vi "ReversedEngineering FilterClassSearch.vi"(0 "dependencyClassPath":path[](array[path]), 2 "LoopIteration":i32, 4 "IgnoreClasses":path[](array[path]), 5 "error in (no error)":errorcluster, 6 "SerachDirs":path[](array[path]), 7 "Only Create this/these classes and its dependencis":bool, 8 "SearchOnlyClasses":bool, 9 "Only analyse this class methods and attributes(False)":bool, 10 "SearchOnlyTopVIs":bool, 11 "SyncOption":T1) -> (14 "dependencyClassPathOut":path[](array[path]), 15 "AnalyseClass":bool, 16 "AnalyseDone":bool, 17 "ClassPathToAnalyse":path, 19 "error out":errorcluster)   [LabVIEW 2012]
uses:
  <resource>/Framework/Providers/Open_GDS/UML/UMLEditor/UMLEditor_SyncOptions.ctl
  <resource>/Framework/Providers/Open_GDS/UML/UmlEditor_class/UmlEditor.lvclass
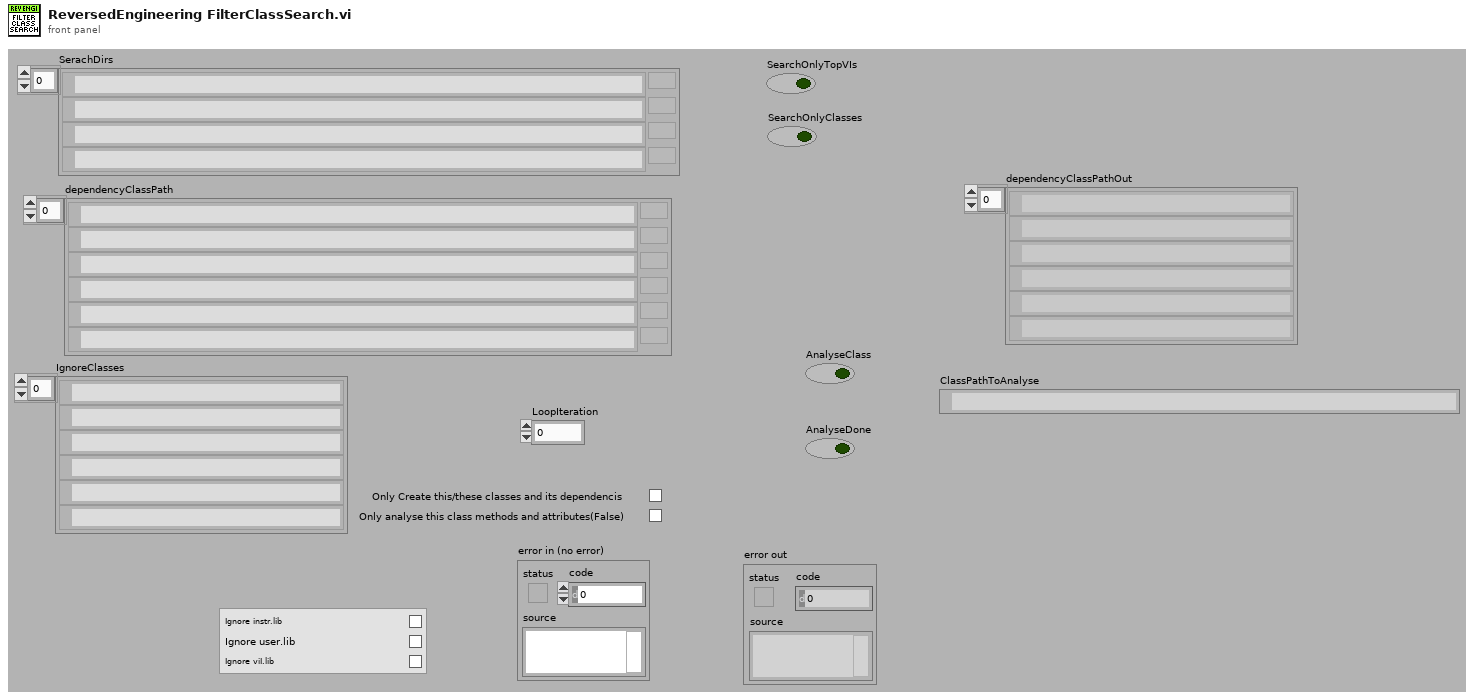
[diagram p1: front panel]
types:
  T1 = typedef "UMLEditor_SyncOptions.ctl" = cluster{"IgnoreInstrLib":bool, "IgnoreUserLib":bool, "IgnoreViLib":bool}
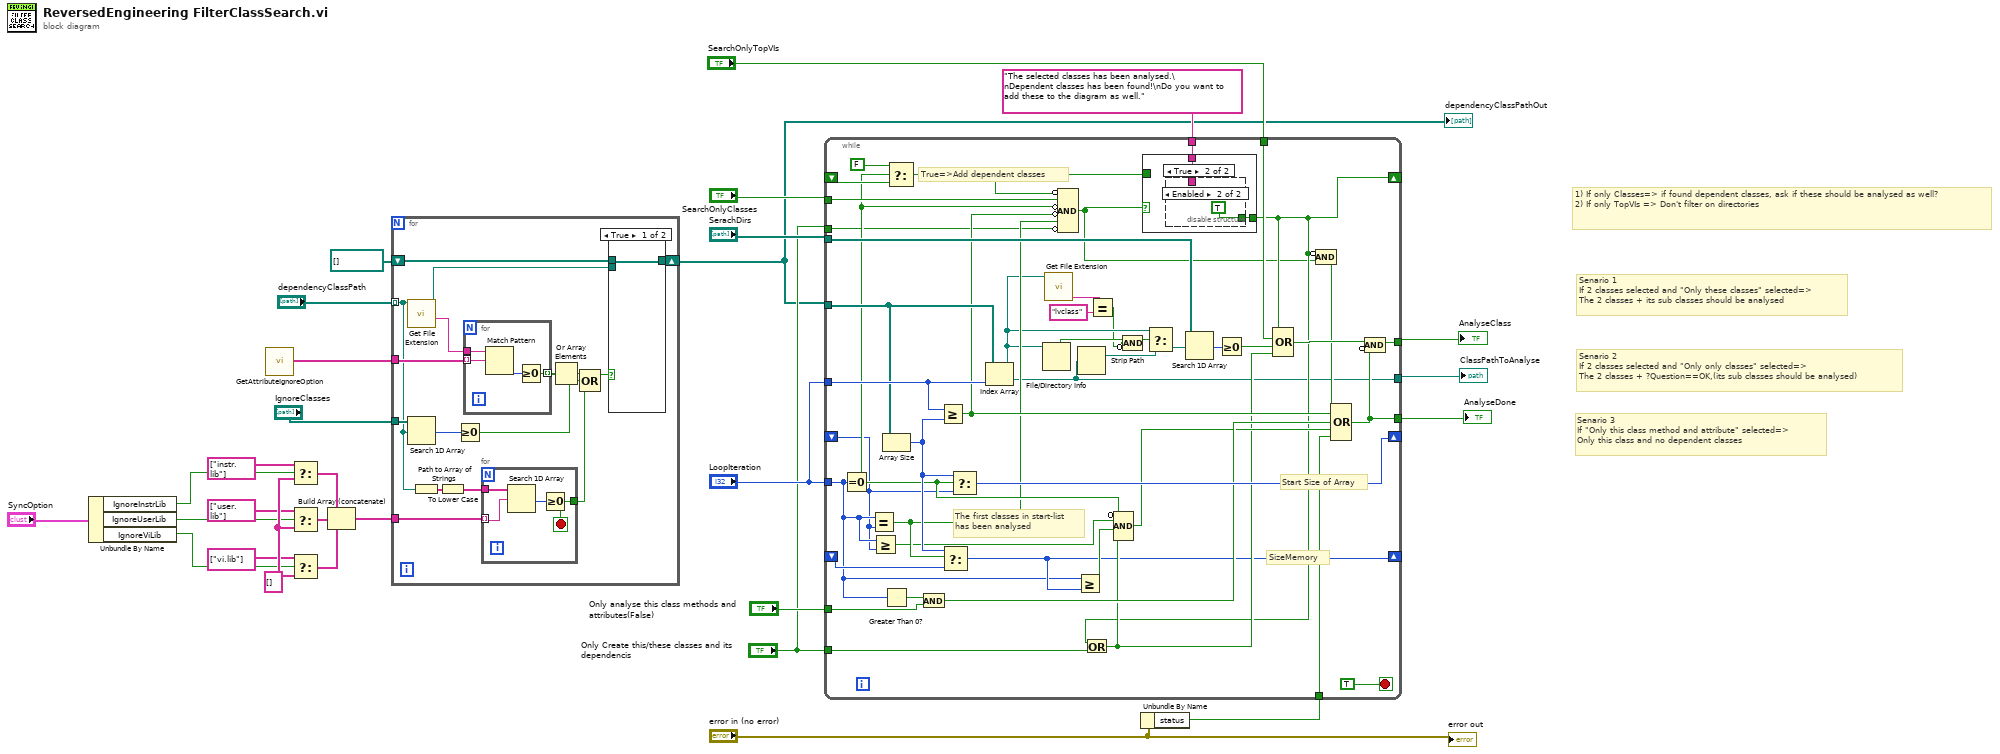
[diagram p0: block diagram]
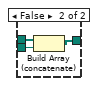
[diagram p2: hidden frame]
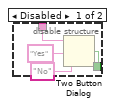
[diagram p4: hidden frame]
diagram:
  w9 = string[] [] ("f")
  # "Senario 3\nIf \"Only this class method and attribute\" selected=>\nOnly this class and no dependent classes"
  # "Senario 2\nIf 2 classes selected and \"Only only classes\" selected=>\nThe 2 classes + ?Question==OK,(its sub classes should be analysed)"
  # "Senario 1\nIf 2 classes selected and \"Only these classes\" selected=>\nThe 2 classes + its sub classes should be analysed"
  # "1) If only Classes=> if found dependent classes, ask if these should be analysed as well?\n2) If only TopVIs => Don't filter on directories"
  n1 = Unbundle By Name("SyncOption") -> ("IgnoreInstrLib"=w11:bool, "IgnoreUserLib"=w6:bool, "IgnoreViLib"=w5:bool)
  n2 = call <resource>:"GetAttributeIgnoreOption.vi"() -> ("ClassesToIgnore"=w16:string[])  [unwired: 1 in, 18 out]
  n3 = Select(t=string[] ["instr.lib"], s=w11, f=w9) -> (s? t:f=w4:string[])
  n4 = Select(t=string[] ["user.lib"], s=w6, f=w9) -> (s? t:f=w3:string[])
  n5 = Select(t=string[] ["vi.lib"], s=w5, f=w9) -> (s? t:f=w2:string[])
  n6 = Build Array (concatenate)(w4, w3, w2) -> (w1:string[])
  n7 = for {
    tunnel: "dependencyClassPath" -> [w34] mode=indexing
    tunnel: w16 -> [w42]
    shift-right: [w43] -> w14
    shift-left: path[] [] -> [w45]
    tunnel: "IgnoreClasses" -> [w39]
    tunnel: w1 -> [w32]
    n8 = call <vilib>:"Get File Extension.vi"("file"=w34) -> ("filename without extension"=w41:string, "dup file"=w44:path)  [unwired: 1 in, 8 out]
    n9 = Search 1D Array(1D array=w39, element=w34) -> (index of element=w38:i32)  [unwired: 1 out]
    n10 = Path to Array of Strings(0:w34) -> (2:w33:string[])  [unwired: 1 out]
    n11 = To Lower Case(string=w33) -> (all lower case string=w31:string[])
    n12 = Greater Or Equal To 0?(x=w38) -> (x >= 0?=w35:bool)
    n13 = for {
      tunnel: w42 -> [w53] mode=indexing
      tunnel: w41 -> [w52]
      tunnel: [w50] -> w40 mode=indexing
      n14 = Match Pattern(string=w52, regular expression=w53) -> (offset past match=w51:i32)  [unwired: 4 out]
      n15 = Greater Or Equal To 0?(x=w51) -> (x >= 0?=w50:bool)
    }
    n16 = for {
      tunnel: w31 -> [w49]
      tunnel: w32 -> [w48] mode=indexing
      tunnel: [w46] -> w30
      stop <- w46 stop-if-true
      n17 = Search 1D Array(1D array=w49, element=w48) -> (index of element=w47:i32)  [unwired: 1 in]
      n18 = Greater Or Equal To 0?(x=w47) -> (x >= 0?=w46:bool)
    }
    n19 = Or Array Elements(Boolean array=w40) -> (logical OR=w36:bool)
    n20 = Compound Arithmetic op=OR(w36, w35, w30) -> (w37:bool)
    n21 = case shown="True" w37 {
      tunnel: w45 -> [w54 w57]
      tunnel: w44 -> [_ w56]
      tunnel: [w54 w55] -> w43
      frame True {
      }
      frame False {
        n22 = Build Array (concatenate)(w57, w56) -> (w55:path[])
      }
    }
  }
  "dependencyClassPathOut" <- w14
  n23 = Unbundle By Name("error in (no error)") -> ("status"=w20:bool)
  n24 = while {
    tunnel: "SerachDirs" -> [w102]
    shift-right: [w101] -> _
    shift-left: _ -> [w73]
    tunnel: "LoopIteration" -> [w74]
    tunnel: "LoopIteration" -> [w95]
    tunnel: w14 -> [w92]
    tunnel: "SearchOnlyTopVIs" -> [w97]
    tunnel: [w62] -> w26
    tunnel: [w94] -> w25
    tunnel: [w93] -> w24
    shift-right: [w76] -> _
    shift-left: _ -> [w78]
    tunnel: "Only analyse this class methods and attributes(False)" -> [w90]
    tunnel: "Only Create this/these classes and its dependencis" -> [w86]
    tunnel: "SearchOnlyClasses" -> [w85]
    shift-right: [w71] -> _
    shift-left: _ -> [w83]
    tunnel: w20 -> [w68]
    tunnel: "The selected classes has been analysed.\nDependent classes has been found!\nDo you want to add these to the diagram as well." ("message") -> [w64]
    tunnel: "Only Create this/these classes and its dependencis" -> [w63]
    stop <- TRUE stop-if-true
    # "True=>Add dependent classes"
    # "The first classes in start-list\nhas been analysed"
    # "SizeMemory"
    # "Start Size of Array"
    n25 = Equal To 0?(x=w74) -> (x = 0?=w77:bool)
    n26 = Equal?(x=w74, y=w73) -> (x = y?=w75:bool)
    n27 = Greater Or Equal?(x=w74, y=w73) -> (x >= y?=w72:bool)
    n28 = Array Size(array=w92) -> (size(s)=w79:i32)
    n29 = Greater Than 0?(x=w74) -> (x > 0?=w91:bool)
    n30 = Select(t=FALSE, s=w77, f=w83) -> (s? t:f=w81:bool)
    n31 = And(x=w91, y=w90) -> (x .and. y?=w89:bool)
    n32 = Greater Or Equal?(x=w95, y=w79) -> (x >= y?=w84:bool)
    n33 = Select(t=w79, s=w75, f=w78) -> (s? t:f=w76:i32)
    n34 = Select(t=w79, s=w77, f=w73) -> (s? t:f=w101:i32)
    n35 = Index Array(array=w92, index=w95) -> (element=w62:path)
    n36 = File/Directory Info(path=w62) -> (directory=w67:bool)  [unwired: 1 in, 6 out]
    n37 = call <vilib>:"Get File Extension.vi"("file"=w62) -> ("lowercase file extension"=w61:string)  [unwired: 1 in, 9 out]
    n38 = Compound Arithmetic op=AND(invert w81, w85, invert w77, invert w84, w75, invert w63) -> (w70:bool)
    n39 = Greater Or Equal?(x=w74, y=w76) -> (x >= y?=w88:bool)
    n40 = Strip Path(path=w62) -> (stripped path=w66:path)  [unwired: 1 out]
    n41 = Equal?(x=w61, y="lvclass") -> (x = y?=w58:bool)
    n42 = Compound Arithmetic op=AND(w67, invert w58) -> (w59:bool)
    n43 = case shown="True" w70 {
      tunnel: [w103 w105] -> w71
      tunnel: w81 -> [w103 _]
      tunnel: w64 -> [_ w104]
      frame False {
      }
      frame True {
        n44 = disable-structure shown="Enabled" {
          disable-tunnel: [w107 TRUE ("t")] -> w105
          disable-tunnel: w104 -> [w106 _]
          frame Disabled {
            n45 = Two Button Dialog(message=w106, 1:"No" ("F button name (\"Cancel\")"), 2:"Yes" ("T button name (\"OK\")")) -> (T button?=w107:bool)
          }
          frame Enabled {
          }
        }
      }
    }
    n46 = Or(x=w71, y=w86) -> (x .or. y?=w80:bool)
    n47 = Compound Arithmetic op=AND(invert w77, w72, w88, w80) -> (w87:bool)
    n48 = Select(t=w62, s=w59, f=w66) -> (s? t:f=w65:path)
    n49 = Search 1D Array(1D array=w102, element=w65) -> (index of element=w99:i32)  [unwired: 1 out]
    n50 = Greater Or Equal To 0?(x=w99) -> (x >= 0?=w98:bool)
    n51 = Compound Arithmetic op=OR(w71, w97, w98, w80) -> (w96:bool)
    n52 = Compound Arithmetic op=AND(invert w71, w70) -> (w69:bool)
    n53 = Compound Arithmetic op=OR(w69, w84, w89, w87, w68) -> (w93:bool)
    n54 = Compound Arithmetic op=AND(w96, invert w93) -> (w94:bool)
  }
  "AnalyseClass" <- w25
  "AnalyseDone" <- w24
  "ClassPathToAnalyse" <- w26
  "error out" <- "error in (no error)"
